vi "NEWHEART.vi"() -> ()   [LabVIEW 2014]
uses:
  <vilib>/Utility/file.llb/Read From Spreadsheet File (string).vi
  <vilib>/Utility/file.llb/Read From Spreadsheet File (DBL).vi
  builds/NEWHEART/NEWHEART/data/ConsoleApplication4.dll
panel:
  in  "File path (.csv)":path=path "D:/new_dataxxx.csv"
  out "Diagnosis code":dbl
  in  "Patient number":u32=1 min=1
  out "Diagnosis":string
  out "Normal":bool
  in  "?":bool
  out "Not Normal":bool
  out "Probability":dbl
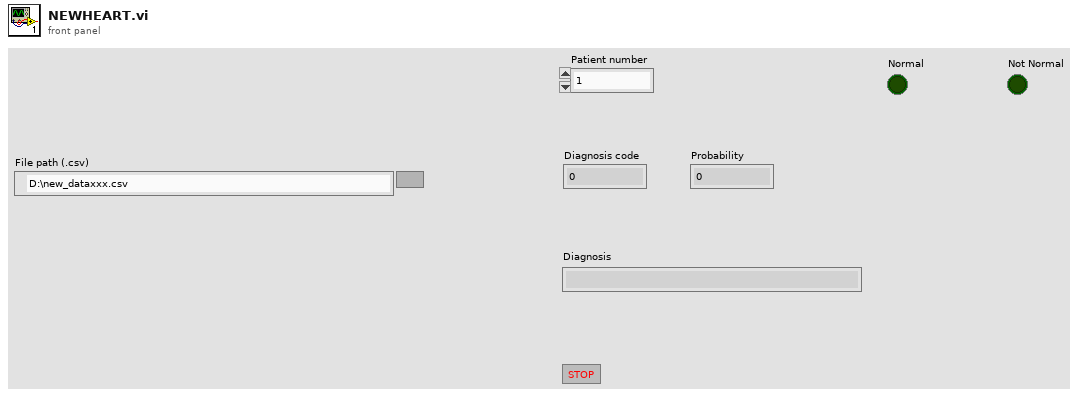
[diagram p1: front panel]
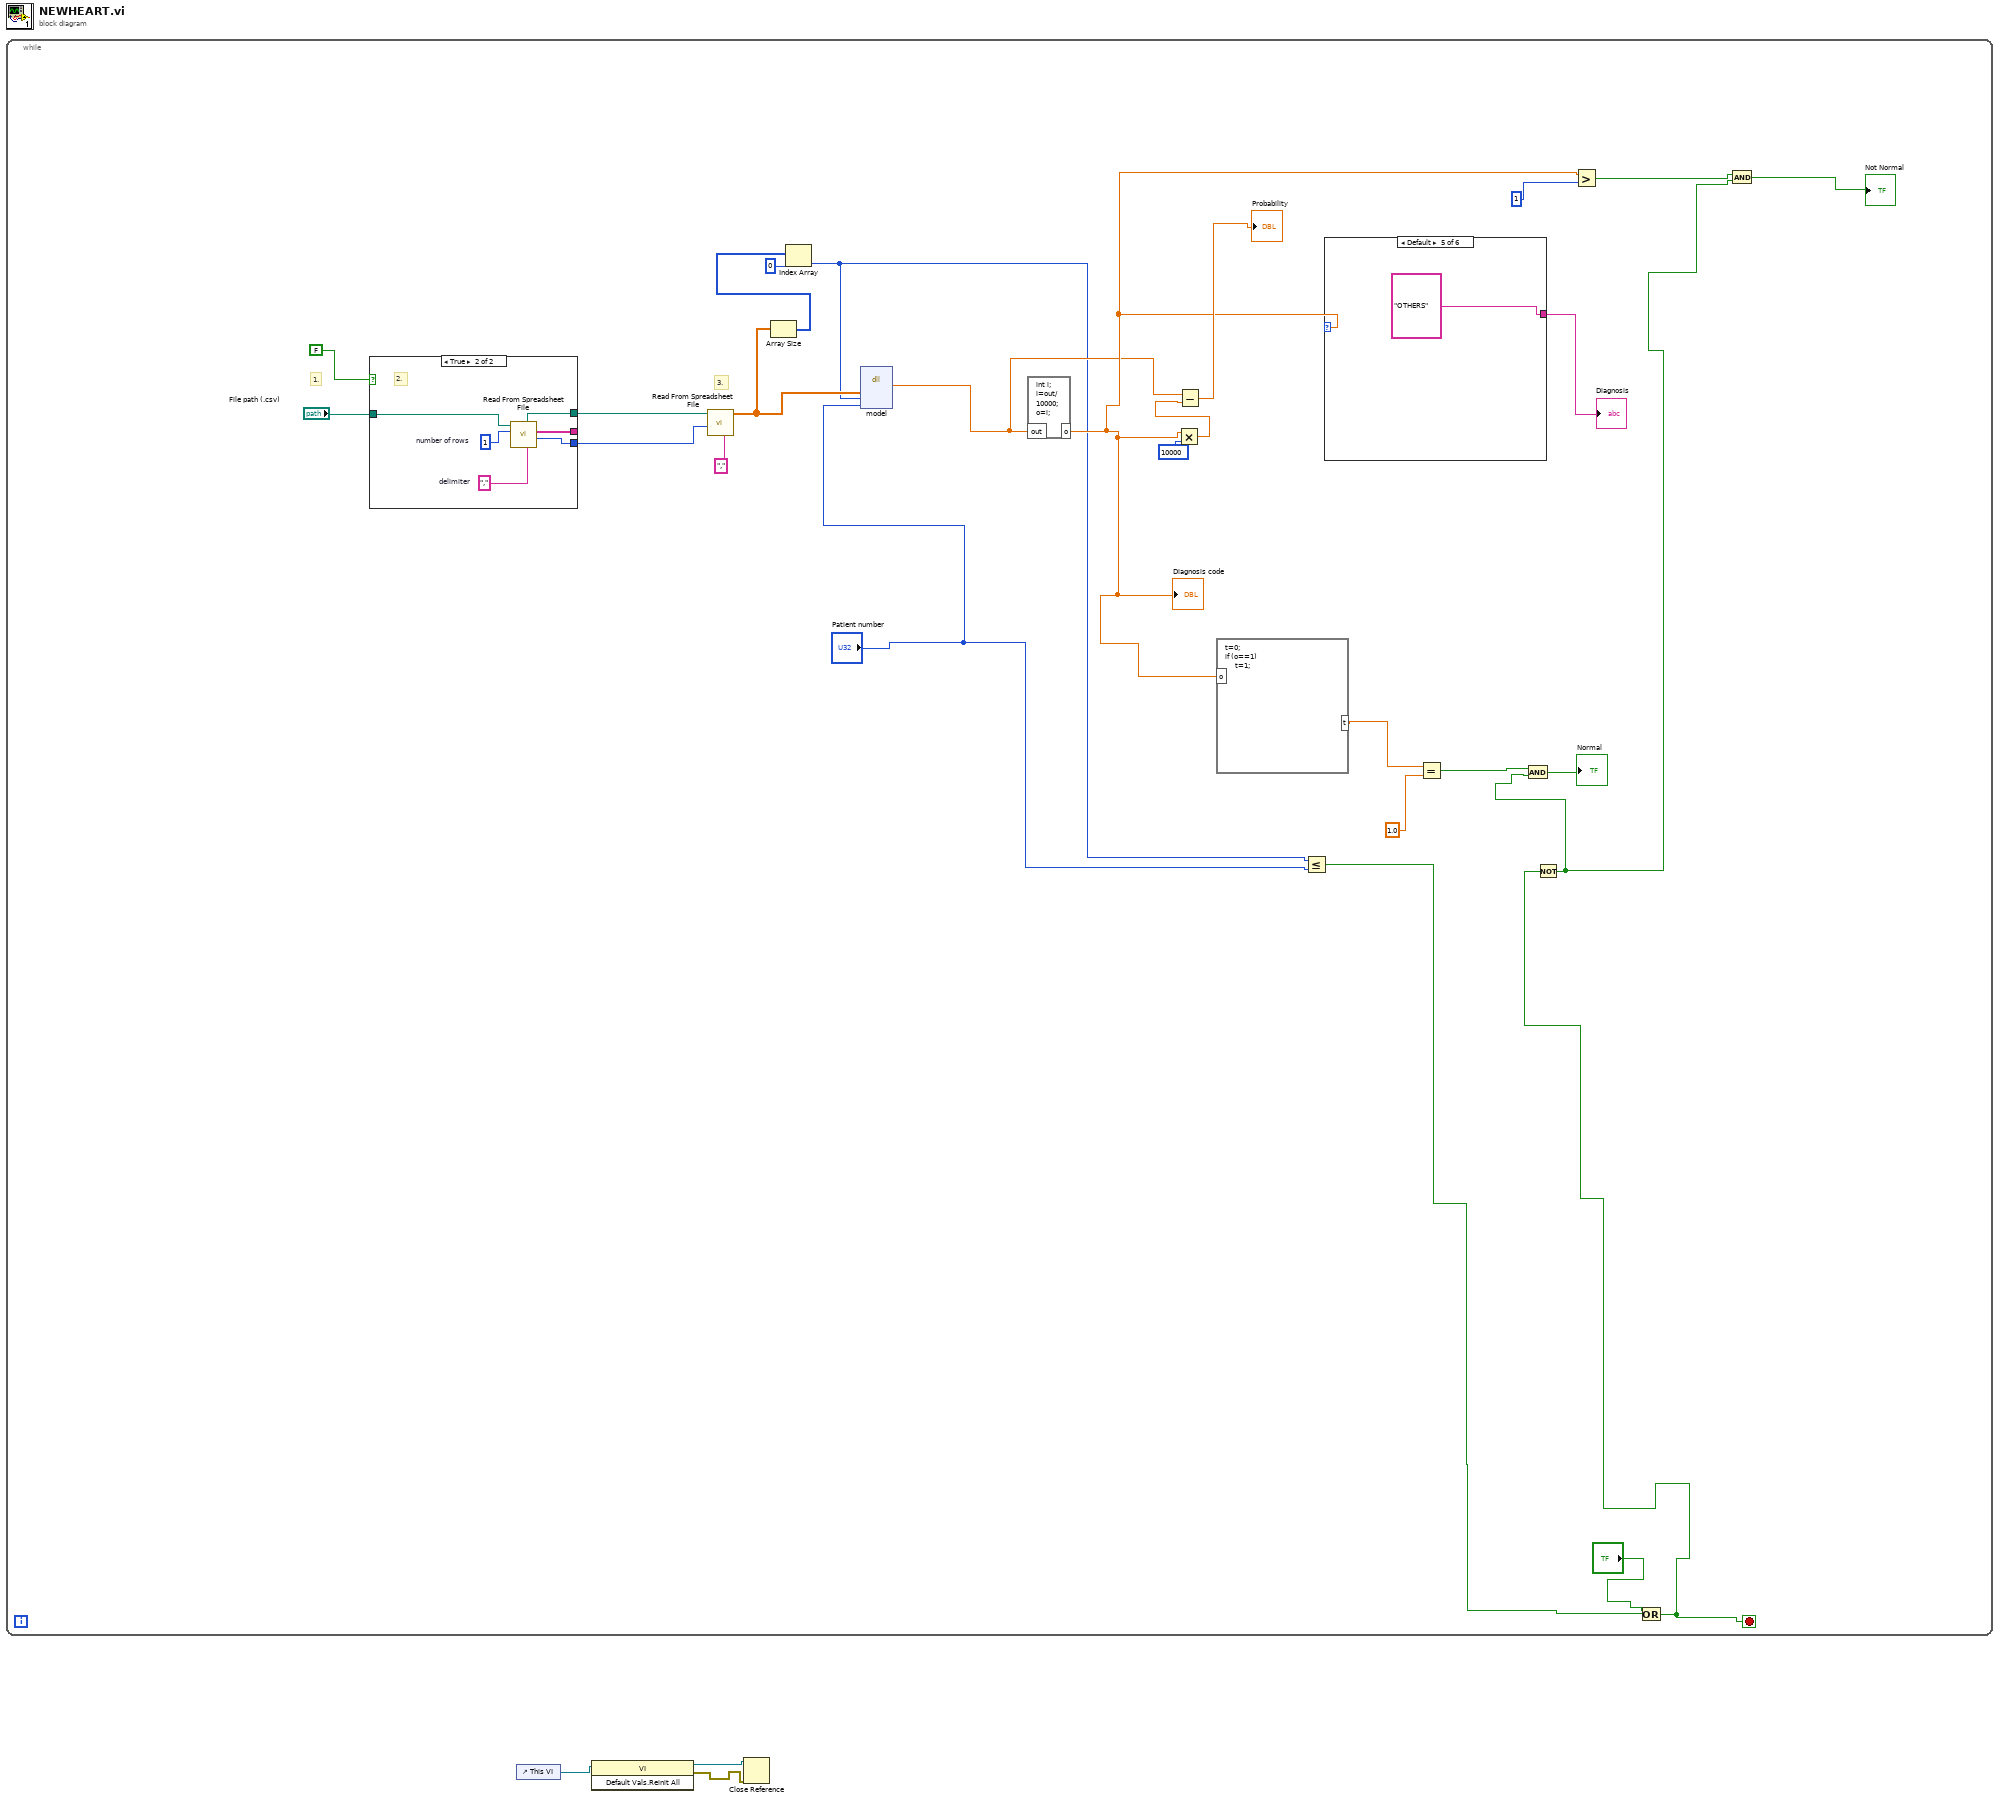
[diagram p0: block diagram]
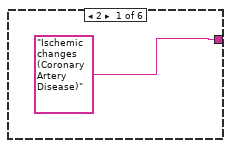
[diagram p2: hidden frame]
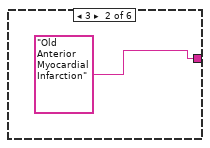
[diagram p3: hidden frame]
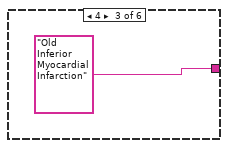
[diagram p4: hidden frame]
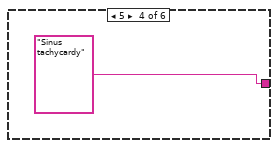
[diagram p5: hidden frame]
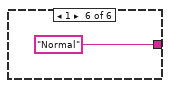
[diagram p6: hidden frame]
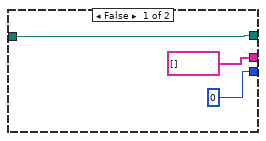
[diagram p7: hidden frame]
diagram:
  n1 = while {
    stop <- w21 stop-if-true
    # "3."
    # "1."
    n2 = case shown="True" FALSE ("My File has Row Headers") {
      tunnel: "File path (.csv)" -> [w37 w45]
      tunnel: [string[] [] ("first row") w43] -> _
      tunnel: [0 ("mark after read (chars.)") w42] -> w26
      tunnel: [w37 w40] -> w28
      frame False {
      }
      frame True {
        w41 = 1  # number of rows
        w44 = ","  # delimiter
        # "2."
        n3 = call-poly <vilib>:"Read From Spreadsheet File.vi"("delimiter (\\t)"=w44, "number of rows (all:-1)"=w41, "file path (dialog if empty)"=w45) -> ("mark after read (chars.)"=w42:i32, "first row"=w43:string[], "new file path (Not A Path if cancelled)"=w40:path)  [unwired: 4 in, 2 out]
      }
    }
    n4 = call-poly <vilib>:"Read From Spreadsheet File.vi"("delimiter (\\t)"="," ("delimiter (\\t)"), "start of read offset (chars.:0)"=w26, "file path (dialog if empty)"=w28) -> ("all rows"=w8:dbl[][])  [unwired: 4 in, 4 out]
    n5 = Array Size(array=w8) -> (size(s)=w13:i32[])
    n6 = Index Array(array=w13, index=0) -> (element=w4:i32)
    n7 = dll-call lib="C:/Users/acer/Desktop/Project/builds/NEWHEART/NEWHEART/data/ConsoleApplication4.dll" fn="model"("A"=w8, "r"=w4, "rowe"="Patient number") -> ("return type"=w5:dbl)  [unwired: 6 in, 2 out]
    n8 = formula code="int i;\ni=out/10000;\no=i;"("out"=w5) -> ("o"=w6:dbl)
    "Diagnosis code" <- w6
    n9 = Multiply(x=w6, y=10000) -> (x*y=w10:dbl)
    n10 = Subtract(x=w5, y=w10) -> (x-y=→"Probability":dbl)
    n11 = formula code="t=0;\nif (o==1)\n     t=1;"("o"=w6) -> ("t"=w15:dbl)
    n12 = Less Or Equal?(x=w4, y="Patient number") -> (x <= y?=w20:bool)
    n13 = case shown="Default" w6 {
      tunnel: ["Ischemic changes (Coronary Artery Disease)" "Old Anterior Myocardial Infarction" "Old Inferior Myocardial Infarction" "Sinus tachycardy" "OTHERS" "Normal"] -> w14
      frame 2 {
      }
      frame 3 {
      }
      frame 4 {
      }
      frame 5 {
      }
      frame Default {
      }
      frame 1 {
      }
    }
    "Diagnosis" <- w14
    n14 = Equal?(x=w15, y=1.0 ("Numeric 2")) -> (x = y?=w24:bool)
    n15 = Greater?(x=w6, y=1) -> (0:w18:bool)
    n16 = Or(x="?", y=w20) -> (x .or. y?=w21:bool)
    n17 = Not(x=w21) -> (.not. x?=w17:bool)
    n18 = And(x=w24, y=w17) -> (x .and. y?=→"Normal":bool)
    n19 = And(x=w18, y=w17) -> (x .and. y?=→"Not Normal":bool)
  }
  n20 = control-ref of="This VI"() -> (w3:refnum<vi>)
  n21 = invoke class="VI" method="Default Vals.Reinit All"(reference=w3) -> (reference out=w2:refnum<vi>, error out=w1:errorcluster)  [unwired: 2 in, 1 out]
  n22 = Close Reference(reference=w2, error in (no error)=w1) -> ()  [unwired: 1 out]
